vi "视屏播放测试.vi"() -> ()   [LabVIEW 2014]
panel:
  out "status":string
  out "windowlessVideo":bool
  out "imageSourceHeight":i32
  out "durationString":string
  out "duration":dbl
  out "attributeCount":i32
  out "versionInfo":string
  in  "停止":bool
  in  "路径":path
  in  "WindowsMediaPlayer":refnum<k7>(container)
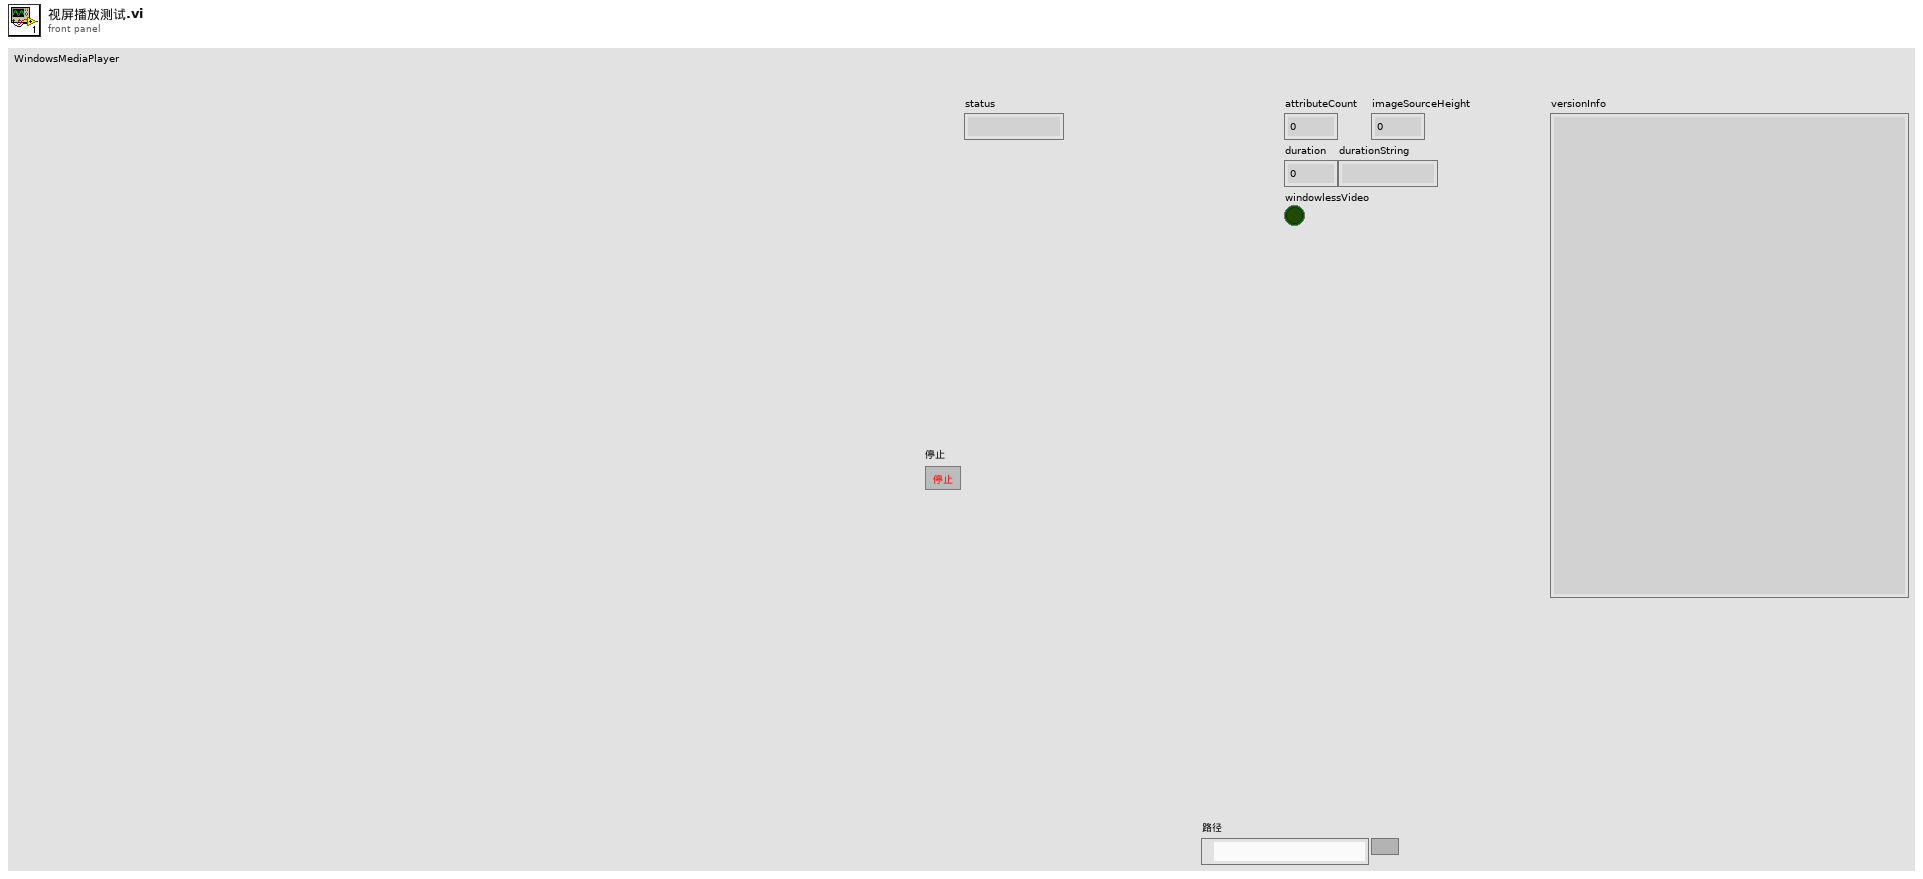
[diagram p1: front panel]
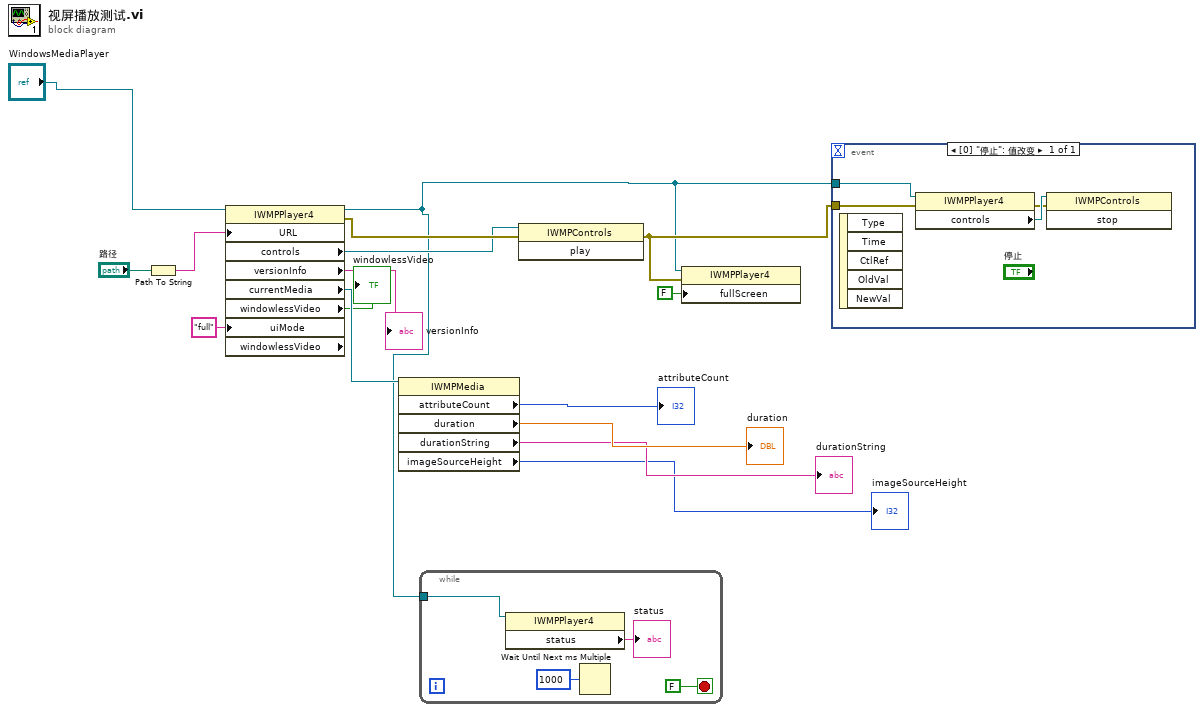
[diagram p0: block diagram]
diagram:
  n1 = Path To String(path="路径") -> (string=w15:string)
  n2 = property class="IWMPPlayer4" props=["URL", "controls", "versionInfo", "currentMedia", "windowlessVideo", "uiMode", "windowlessVideo"](reference="WindowsMediaPlayer", "URL"=w15, "uiMode"="full") -> (reference out=w1:refnum<k7>, error out=w14:errorcluster, "controls"=w2:refnum<k7>, "versionInfo"=→"versionInfo":string, "currentMedia"=w9:refnum<k7>, "windowlessVideo"=→"windowlessVideo":bool)  [unwired: 1 in, 1 out]
  n3 = property class="IWMPMedia"(reference=w9) -> ("attributeCount"=→"attributeCount":i32, "duration"=→"duration":dbl, "durationString"=→"durationString":string, "imageSourceHeight"=→"imageSourceHeight":i32)  [unwired: 1 in, 2 out]
  n4 = while {
    tunnel: w1 -> [w19]
    stop <- FALSE stop-if-true
    n5 = property class="IWMPPlayer4"(reference=w19) -> ("status"=→"status":string)  [unwired: 1 in, 2 out]
    n6 = Wait Until Next ms Multiple(millisecond multiple=u32 1000 ("毫秒倍数")) -> ()  [unwired: 1 out]
  }
  n7 = invoke class="IWMPControls" method="play"(reference=w2, error in=w14) -> (error out=w12:errorcluster)  [unwired: 1 in, 2 out]
  n8 = property class="IWMPPlayer4"(reference=w1, error in=w12, "fullScreen"=FALSE) -> ()  [unwired: 2 out]
  n9 = event shown="[0] \"停止\": 值改变" {
    selector: _ -> [_]
    dyn-events: _ -> [_]
    timeout: _ -> [_]
    tunnel: w1 -> [w24]
    tunnel: w12 -> [w23]
    event "停止": Value Change {
      n10 = event-data() -> ()  [unwired: 1 in, 5 out]
      n11 = property class="IWMPPlayer4"(reference=w24, error in=w23) -> (error out=w21:errorcluster, "controls"=w22:refnum<k7>)  [unwired: 1 out]
      n12 = invoke class="IWMPControls" method="stop"(reference=w22, error in=w21) -> ()  [unwired: 1 in, 3 out]
    }
  }
